vi "ZY-3100 mode convert.vi"(11 "测试机台选择":tag) -> (0 "错误输出":errorcluster, 2 "测试机台选择":tag, 3 "引用句柄输出":refnum<k21>)   [LabVIEW 2019]
uses:
  <vilib>/VirtualBench/VirtualBench.lvlib
panel:
  in  "Data":bool[](array[boolean])=[TRUE]
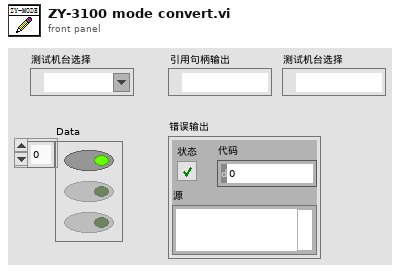
[diagram p1: front panel]
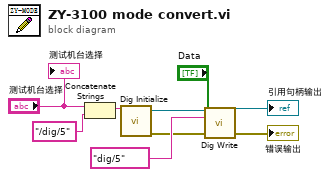
[diagram p0: block diagram]
diagram:
  n1 = Concatenate Strings("测试机台选择", "/dig/5" ("字符串")) -> (w4:string)
  n2 = call <vilib>:"Dig Initialize.vi"("Lines"=w4) -> ("Instrument Handle Out"=w7:refnum<k21>, "Error Out"=w5:errorcluster)  [unwired: 13 in]
  n3 = call <vilib>:"Dig Write.vi"("Instrument Handle In"=w7, "Lines"=tag "dig/5", "Data"="Data", "Error In"=w5) -> ("Instrument Handle Out"=→"引用句柄输出":refnum<k21>, "Error Out"=→"错误输出":errorcluster)  [unwired: 10 in]
  "测试机台选择" <- "测试机台选择"
